vi "GetImage.vi"(8 "error in (no error)":errorcluster, 11 "Image in":refnum<class "Image.lvclass">) -> (0 "error out":errorcluster, 2 "Image":T1, 3 "Image out":refnum<class "Image.lvclass">)   [LabVIEW 2012, in "Image.lvclass"]
uses:
  Image.lvclass
  <vilib>/vision/Image Controls.llb/IMAQ Image.ctl
  Image.lvclass/Image.ctl
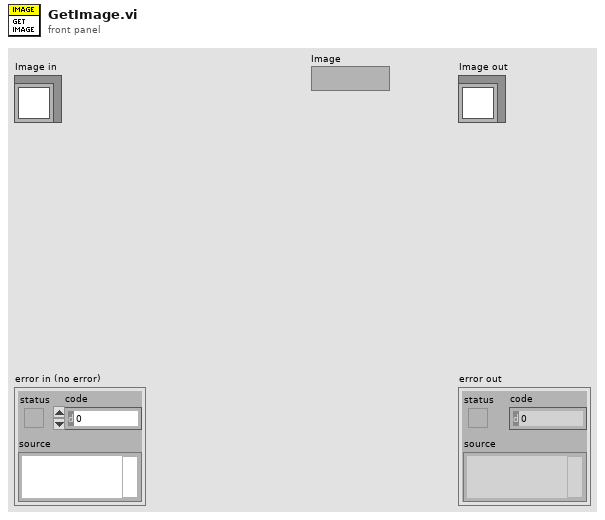
[diagram p1: front panel]
types:
  T1 = typedef "IMAQ Image.ctl" = refnum<image>
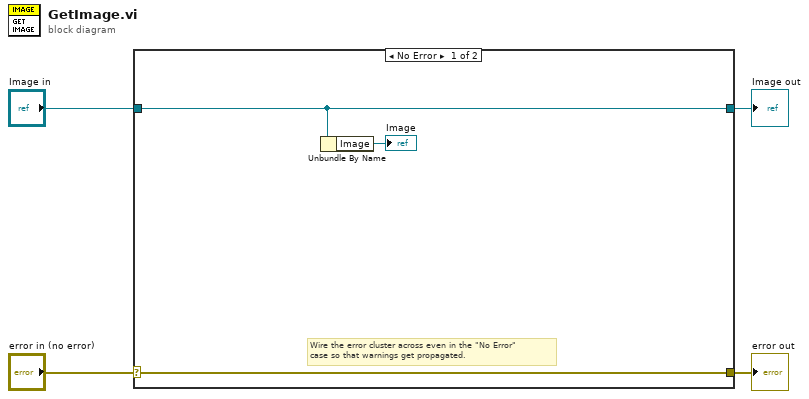
[diagram p0: block diagram]
diagram:
  n1 = case shown="No Error" "error in (no error)" {
    selector: "error in (no error)" -> [w7 w9]
    tunnel: [w7 w9] -> w3
    tunnel: [w6 w8] -> w1
    tunnel: "Image in" -> [w6 w8]
    frame No Error {
      # "Wire the error cluster across even in the \"No Error\"\ncase so that warnings get propagated."
      n2 = Unbundle By Name(w6) -> ("Image"=→"Image":T1)
    }
    frame Error {
    }
  }
  "error out" <- w3
  "Image out" <- w1
